vi "RQS Wait VISA.vi"() -> ()   [LabVIEW 2018]
uses:
  <vilib>/Instr/_visa.llb/Select Event Type.ctl
panel:
  out "Event Type":T1=1073684491 items=["Service Request"=1073684491, "Trigger"=3221168138, "Clear"=1073684493, "VXI Signal"=1073684512, "VXI/VME Interrupt"=3221168161, "VXI/VME Sysfail"=1073684509, "VXI/VME Sysreset"=1073684510, "GPIB CIC"=1073684498, "GPIB Talk"=1073684499, "GPIB Listen"=1073684500, "PXI Interrupt"=1073684514, "Serial Break"=1073684515, "Serial TermChar"=1073684516, "Serial CTS"=1073684521, "Serial DSR"=1073684522, "Serial DCD"=1073684524, "Serial RI"=1073684526, "Serial Character"=1073684533, "USB Interrupt"=1073684535, "All Enabled"=1073709055]
  out "error out":errorcluster
  in  "error in (no error)":errorcluster
  out "VISA resource name out":refnum<visa-resource-name>
  out "status byte":u16
  in  "VISA Session":refnum<visa-resource-name>
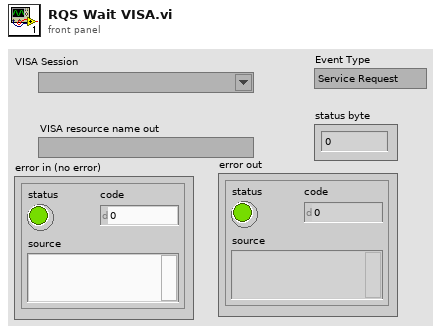
[diagram p1: front panel]
types:
  T1 = typedef "Select Event Type.ctl" = u32
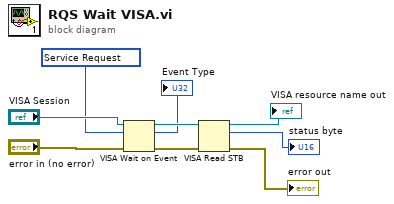
[diagram p0: block diagram]
diagram:
  w6 = T1 1073684491 items=["Service Request"=1073684491, "Trigger"=3221168138, "Clear"=1073684493, "VXI Signal"=1073684512, "VXI/VME Interrupt"=3221168161, "VXI/VME Sysfail"=1073684509, "VXI/VME Sysreset"=1073684510, "GPIB CIC"=1073684498, "GPIB Talk"=1073684499, "GPIB Listen"=1073684500, "PXI Interrupt"=1073684514, "Serial Break"=1073684515, "Serial TermChar"=1073684516, "Serial CTS"=1073684521, "Serial DSR"=1073684522, "Serial DCD"=1073684524, "Serial RI"=1073684526, "Serial Character"=1073684533, "USB Interrupt"=1073684535, "All Enabled"=1073709055] ("Event Type")
  n1 = VISA Wait on Event(8:"error in (no error)", 10:w6, 11:"VISA Session") -> (0:w4:errorcluster, 2:→"Event Type":u32, 3:w5:refnum<visa-resource-name>)  [unwired: 2 in, 1 out]
  n2 = VISA Read STB(8:w4, 11:w5) -> (0:→"error out":errorcluster, 2:→"status byte":u16, 3:→"VISA resource name out":refnum<visa-resource-name>)
